vi "ReadHandleOut.vi"(8 "error in (no error)":errorcluster, 11 "object in":refnum<class "Hamamatsu.lvclass">) -> (0 "error out":errorcluster, 2 "Handle out":u32, 3 "object out":refnum<class "Hamamatsu.lvclass">)   [LabVIEW 2019, in "Hamamatsu.lvclass"]
uses:
  Hamamatsu.lvclass
  Hamamatsu.lvclass/Hamamatsu.ctl
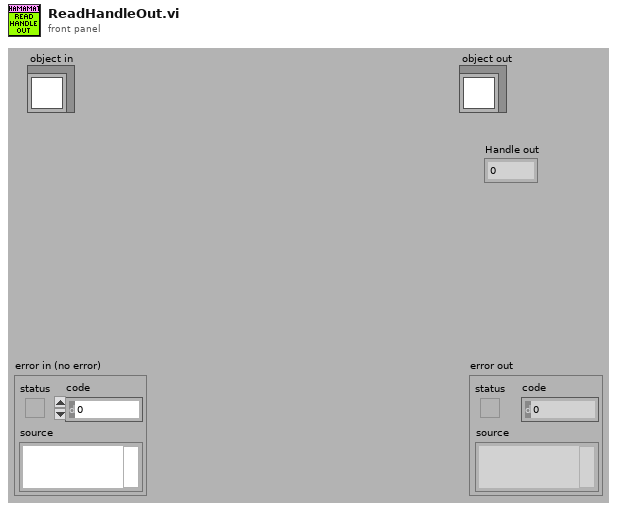
[diagram p1: front panel]
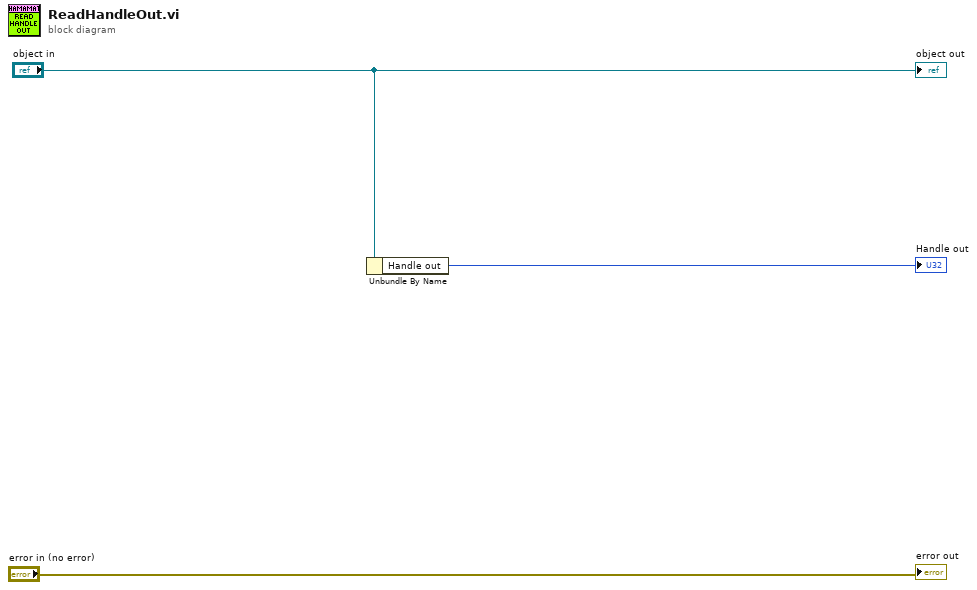
[diagram p0: block diagram]
diagram:
  n1 = Unbundle By Name("object in") -> ("Handle out"=→"Handle out":u32)
  "error out" <- "error in (no error)"
  "object out" <- "object in"
